vi "FFT Measurement test.vi"   [LabVIEW 2014]
uses:
  <vilib>/Platform/TimedLoop/XDataNode/timing_clust.ctl
  <vilib>/Platform/TimedLoop/XDataNode/nitl_modes.ctl
  <vilib>/Platform/TimedLoop/XDataNode/wakeup.ctl
  <vilib>/rvi/Analysis/measure/FFT/simModelSupport/niFPGA FFT Streaming Sim Properties.ctl
  <vilib>/rvi/Analysis/measure/FFT/simModelSupport/niFPGA FFT Sim Stream Group Properties.ctl
  <vilib>/rvi/Analysis/measure/FFT/simModelSupport/niFPGA FFT Sim Types.ctl
  <vilib>/rvi/Analysis/measure/FFT/simModelSupport/niFpgaFFTSimArithmeticProperties.ctl
  <vilib>/rvi/Analysis/measure/FFT/simModelSupport/niFpgaFFTSimDfxp.ctl
  <vilib>/fxp/LVFixedPointQuantizationPolicyTypeDef.ctl
  <vilib>/rvi/Analysis/measure/FFT/XNode/niFpgaFFTButterflyDelays.ctl
  <vilib>/rvi/Emulation/niFpgaSctlEmulationGetInTimedLoop.vi
  <vilib>/rvi/Emulation/niFpgaEmulationReportErrorSimple.vi
  <vilib>/rvi/Emulation/niFpgaGetClockAttributes.vi
  <vilib>/rvi/Emulation/niFpgaCriticalErrorInLSC.vi
  <vilib>/rvi/Memory/Memory_Emulation/nirvimemoryFastEmulation.vi
  <vilib>/rvi/Memory/Memory_Emulation/nirvimemoryEmulation.vi
  <vilib>/rvi/Emulation/niFpgaEmulationIsFPGAContextNoSignature.vi
  <vilib>/rvi/DataTransferAndStorage/Container/Common/niFpgaContainerGetUniqueNameForEmu.vi
  <vilib>/rvi/Emulation/niFpgaProcessEmulError.vi
  <vilib>/rvi/errors/nirviReportUnexpectedCaseInternalError (U32).vi
  <vilib>/rvi/errors/niFpgaSetErrorForExecOnDevCompSimple.vi
  <vilib>/rvi/eio/common/nirviEmuReportErrorAndStop.vi
  <vilib>/rvi/FIFO/Fifo_Resource/nirvififoEmulationSetSize.vi
  <vilib>/rvi/FIFO/Fifo_Resource/nirviFifoEmulationQueueMgr.vi
  <instcachedir>/0/nirviFifoEmulationQueueMgr_E5CAEC123FF24DC58D834DCA3CDAA9B5.lvgen/nirviFifoEmulationQueueMgr_E5CAEC123FF24DC58D834DCA3CDAA9B5_004.vi
  <vilib>/rvi/FIFO/Fifo_Resource/nirvififoEmulationDetermineInputValidOut.vi
  <vilib>/rvi/FIFO/Fifo_Resource/nirvififoEmulationCreateLock.vi
  <vilib>/rvi/FIFO/Fifo_Resource/nirvififoEmulationObtainLock.vi
  <vilib>/rvi/FIFO/Fifo_Resource/nirvififoEmulationReleaseLock.vi
  <vilib>/rvi/occurrence/nirviWaitOnOccurrenceBase.vi
  <vilib>/rvi/errors/nirviReportUnexpectedCaseInternalError.vi
  <vilib>/Utility/error.llb/Clear Errors.vi
  <vilib>/rvi/interface/RandomDataEmulation/niFpgaRandomDataHandleErrors.vi
  <vilib>/rvi/Analysis/measure/FFT/simModelSupport/niFpgaFFTSimModelStreamingCore.vi
  <vilib>/rvi/eio/common/nirviEmuTemplateMethod_errors.vi
  <vilib>/Platform/TimedLoop/XDataNode/XDataNode.xnode
  <vilib>/rvi/DataTransferAndStorage/Container/XNode/niFpgaContainer.xnode
  <vilib>/rvi/FIFO/Fifo_Resource/nirvififoEmulationWrite.vi
  <vilib>/rvi/FIFO/Fifo_Resource/nirvififoEmulationRead.vi
  <vilib>/rvi/interface/RandomDataEmulation/nirviRandomDataFpgaReadWriteTemplate.vi
  <vilib>/rvi/Analysis/measure/FFT/XNode/niFpgaFFT.xnode
  <vilib>/eio/EIOMethodNode/EIOMethodNode.xnode
  <vilib>/Platform/TimedLoop/XDataNode/XDNodeRunTimeDep.lvlib
types:
  T1 = typedef "XDNodeRunTimeDep.lvlib/timing_clust.ctl" = cluster{"Expected End [f-1]":u64, "Actual End [f-1]":u64, "Finished Late? [f-1]":bool, "Expected End [i-1]":u64, "Actual End [i-1]":u64, "Finished Late? [i-1]":bool, "Expected Start [i]":u64, "Actual Start [i]":u64, "Expected Start [f]":u64, "Actual Start [f]":u64, "Source Name":string, "Structure Name":string, "Period":i64, "Deadline":i64, "Offset":i64, "Start":i64, "Priority":i32, "Timeout":i32, "Mode":T2, "Wakeup Reason":T3, "Error":errorcluster, "Source Type":string, "Secondary Source Type":string, "Global End Time":u64, "Global Start Time":u64, "Frame Duration":u64, "Iteration Duration":u64, "Assigned CPU":i32, "I/O Scan Engine Mode":u32}
  T2 = typedef "XDNodeRunTimeDep.lvlib/nitl_modes.ctl" = enum32{"No Change", "Process missed periods, maintain original phase", "Discard missed periods, maintain original phase", "Process missed periods, ignore original phase", "Discard missed periods, ignore original phase"}
  T3 = typedef "XDNodeRunTimeDep.lvlib/wakeup.ctl" = enum32{"Normal", "Aborted", "Asynchronous wakeup", "Timing source error", "Timed loop error", "Timeout"}
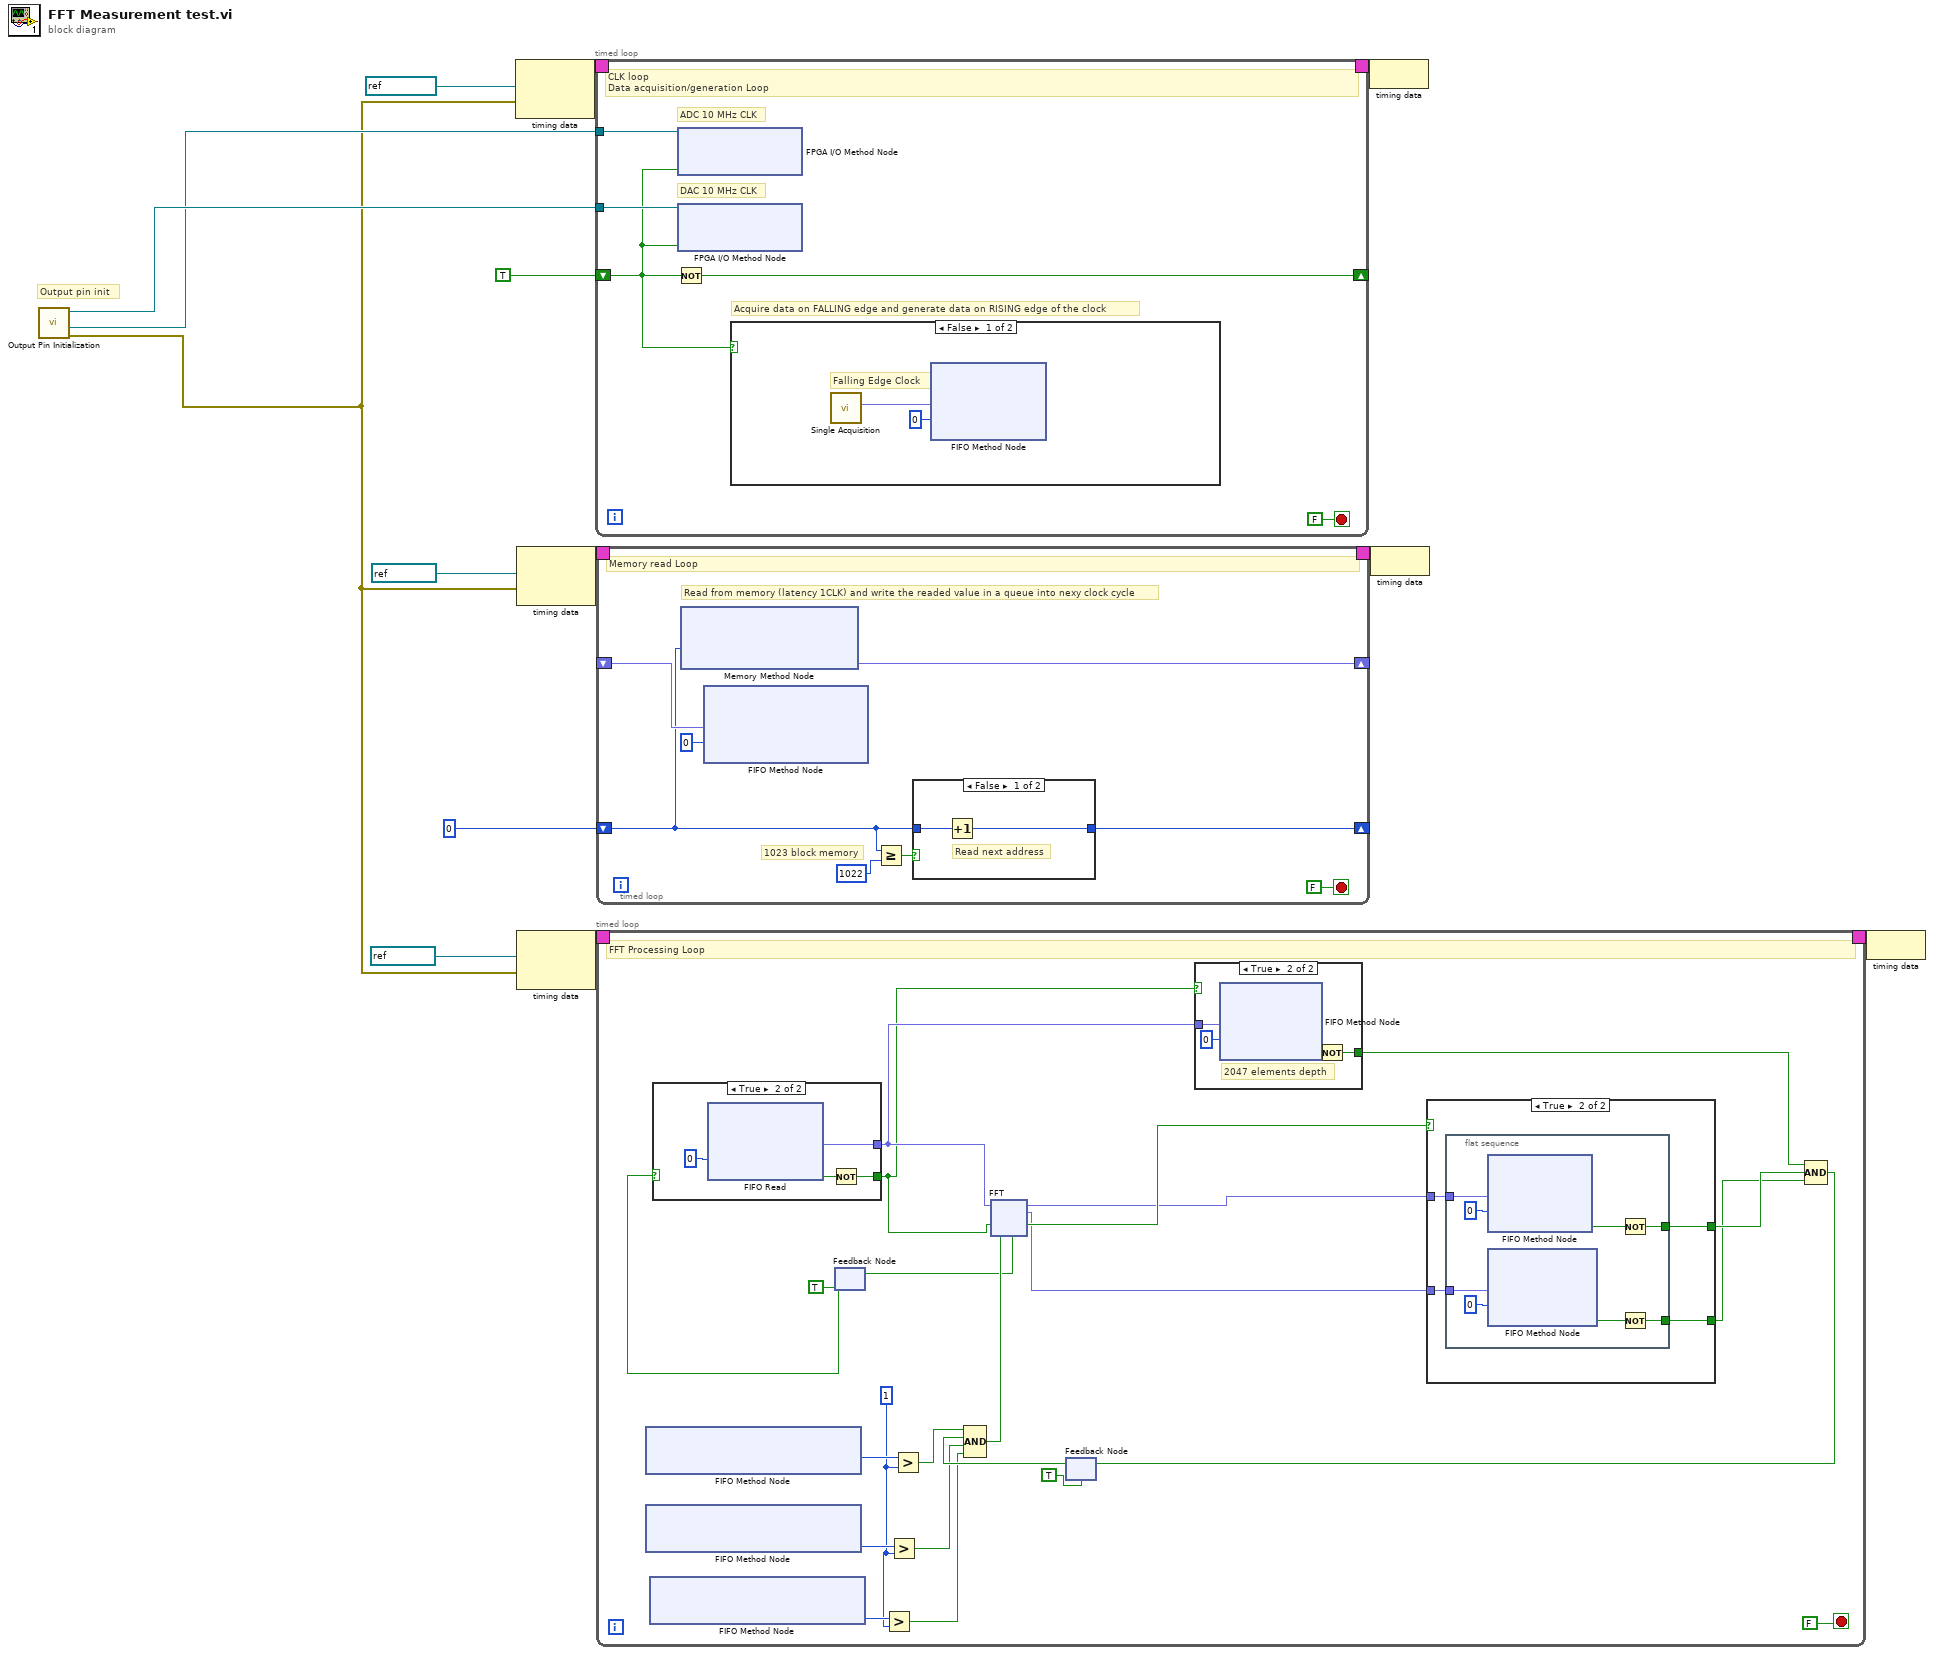
[diagram p0: block diagram]
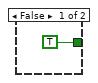
[diagram p2: hidden frame]
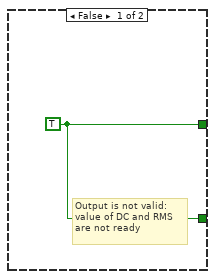
[diagram p3: hidden frame]
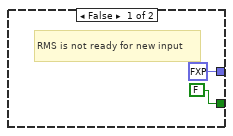
[diagram p4: hidden frame]
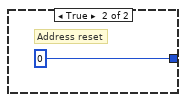
[diagram p5: hidden frame]
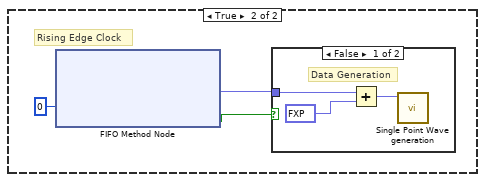
[diagram p6: hidden frame]
diagram:
  # "Output pin init"
  n1 = call "Output Pin Initialization.vi"() -> ("error out"=w1:errorcluster, "I/O Out Clock DAC (pin16)"=w2:refnum<k21>, "I/O Out Clock ADC (pin17)"=w3:refnum<k21>)  [unwired: 8 in]
  n2 = node-c288(refnum<k21> "100MHz" ("Source Name"), w1) -> (w14:T1)
  n3 = node-c288(refnum<k21> "50MHz" ("Source Name"), w1) -> (w12:T1)
  n4 = node-c288(refnum<k21> "50MHz" ("Source Name"), w1) -> (w10:T1)
  n5 = timed-loop {
    timing: w14 -> [_]
    timing-out: [_] -> w13
    shift-right: [w17] -> _
    shift-left: TRUE -> [w15]
    tunnel: w2 -> [w19]
    tunnel: w3 -> [w16]
    stop <- FALSE stop-if-true
    # "DAC 10 MHz CLK"
    # "Acquire data on FALLING edge and generate data on RISING edge of the clock"
    # "ADC 10 MHz CLK"
    # "CLK loop\nData acquisition/generation Loop"
    n6 = Not(x=w15) -> (.not. x?=w17:bool)
    n7 = xnode "FPGA I/O Method Node"("FPGA I/O In"=w19, "Data"=w15) -> ()  [unwired: 1 out]
    n8 = xnode "FPGA I/O Method Node"("FPGA I/O In"=w16, "Data"=w15) -> ()  [unwired: 1 out]
    n9 = case shown="False" w15 {
      frame False {
        # "Falling Edge Clock"
        n10 = call "Single Acquisition.vi"() -> ("Out"=w20:fxp<+/-,12,12>)  [unwired: 10 in, 1 out]
        n11 = xnode ("FIFO Method Node")("Element"=w20, "Timeout"=0) -> ()  [unwired: 1 in, 2 out]
      }
      frame True {
        # "Rising Edge Clock"
        n12 = xnode ("FIFO Method Node")("Timeout"=0) -> ("Element"=w22:fxp<+/-,12,12>, "Timed Out?"=w23:bool)  [unwired: 1 in, 1 out]
        n13 = case shown="False" w23 {
          tunnel: w22 -> [w27 _]
          frame False {
            # "Data Generation"
            n14 = Add(x=w27, y=fxp<+,12,12> 2048.0) -> (x+y=w25:fxp<+/-,14,14>)
            n15 = call "Single Point Wave generation.vi"("Data To Write"=w25) -> ()  [unwired: 10 in, 1 out]
          }
          frame True {
            # "FPGA memory slow"
          }
        }
      }
    }
  }
  n16 = timed-loop {
    timing: w12 -> [_]
    timing-out: [_] -> w11
    shift-right: [w37] -> _
    shift-left: _ -> [w33]
    shift-right: [w34] -> _
    shift-left: u32 0 -> [w30]
    stop <- FALSE stop-if-true
    # "1023 block memory"
    # "Read from memory (latency 1CLK) and write the readed value in a queue into nexy clock cycle"
    # "Memory read Loop"
    n17 = xnode ("Memory Method Node")("Address"=w30) -> ("Data"=w37:fxp<+/-,12,12>)  [unwired: 1 in, 1 out]
    n18 = xnode ("FIFO Method Node")("Element"=w33, "Timeout"=0) -> ()  [unwired: 1 in, 2 out]
    n19 = Greater Or Equal?(x=w30, y=u32 1022) -> (x >= y?=w35:bool)
    n20 = case shown="False" w35 {
      tunnel: w30 -> [w39 _]
      tunnel: [w38 u32 0] -> w34
      frame False {
        # "Read next address"
        n21 = Increment(x=w39) -> (x+1=w38:u32)
      }
      frame True {
        # "Address reset"
      }
    }
  }
  n22 = timed-loop {
    timing: w10 -> [_]
    timing-out: [_] -> w9
    stop <- FALSE stop-if-true
    w45 = u32 1 ("y")
    # "FFT Processing Loop"
    n23 = xnode ("FIFO Method Node")() -> ("Number of Elements to Write"=w62:u32)  [unwired: 1 in, 1 out]
    n24 = xnode ("FIFO Method Node")() -> ("Number of Elements to Write"=w47:u32)  [unwired: 1 in, 1 out]
    n25 = xnode ("FIFO Method Node")() -> ("Number of Elements to Write"=w46:u32)  [unwired: 1 in, 1 out]
    n26 = feedback #1(TRUE ("ready for input")) -> (w65:bool)
    n27 = case shown="True" w65 {
      tunnel: [FALSE w115] -> w57
      tunnel: [fxp<+/-,12,12> 0.0 ("Element") w112] -> w58
      frame False {
        # "RMS is not ready for new input"
      }
      frame True {
        n28 = xnode ("FIFO Read")("Timeout"=0) -> ("Element"=w112:fxp<+/-,12,12>, "Timed Out?"=w114:bool)  [unwired: 1 in, 1 out]
        n29 = Not(x=w114) -> (.not. x?=w115:bool)
      }
    }
    n30 = Greater?(x=w46, y=w45) -> (0:w43:bool)
    n31 = Greater?(x=w47, y=w45) -> (0:w44:bool)
    n32 = Greater?(x=w62, y=w45) -> (0:w61:bool)
    n33 = feedback #2(TRUE) -> (w59:bool)
    n34 = Compound Arithmetic op=AND(w61, w59, w44, w43) -> (w56:bool)
    n35 = xnode "FFT"("real data in"=w58, "input valid"=w57, "ready for output"=w56) -> ("ready for input"=w55:bool, "real data out"=w53:fxp<+/-,21,21>, "imaginary data out"=w52:fxp<+/-,21,21>, "output valid"=w54:bool)  [unwired: 2 in, 1 out]
    n36 = feedback-in #1(w55) -> ()
    n37 = case shown="True" w57 {
      tunnel: w58 -> [_ w96]
      tunnel: [TRUE w93] -> w51
      frame False {
      }
      frame True {
        # "2047 elements depth"
        n38 = xnode ("FIFO Method Node")("Element"=w96, "Timeout"=0) -> ("Timed Out?"=w94:bool)  [unwired: 1 in, 1 out]
        n39 = Not(x=w94) -> (.not. x?=w93:bool)
      }
    }
    n40 = case shown="True" w54 {
      tunnel: w53 -> [_ w101]
      tunnel: w52 -> [_ w100]
      tunnel: [w97 w99] -> w50
      tunnel: [w97 w98] -> w49
      frame False {
        w97 = TRUE
        # "Output is not valid:\nvalue of DC and RMS\nare not ready"
      }
      frame True {
        n41 = flat-sequence {
          tunnel: w101 -> [w109]
          tunnel: w100 -> [w108]
          tunnel: [w103] -> w99
          tunnel: [w102] -> w98
          frame #0 {
            n42 = xnode ("FIFO Method Node")("Element"=w109, "Timeout"=0) -> ("Timed Out?"=w104:bool)  [unwired: 1 in, 1 out]
            n43 = xnode ("FIFO Method Node")("Element"=w108, "Timeout"=0) -> ("Timed Out?"=w105:bool)  [unwired: 1 in, 1 out]
            n44 = Not(x=w104) -> (.not. x?=w103:bool)
            n45 = Not(x=w105) -> (.not. x?=w102:bool)
          }
        }
      }
    }
    n46 = Compound Arithmetic op=AND(w51, w50, w49) -> (w48:bool)
    n47 = feedback-in #2(w48) -> ()
  }
  n48 = node-c288(w13) -> ()
  n49 = node-c288(w11) -> ()
  n50 = node-c288(w9) -> ()
